vi "ProgressCmdResponse.vi"(6 "error in (no error)":errorcluster, 8 "FW Message Length":i32, 9 "FW Message ID":i32, 10 "Command for FW upgrade":string="1||1||1||AC.bin||PC.bin||SC.bin", 11 "connection ID control":refnum<k5>) -> (0 "data out":string, 1 "error out":errorcluster, 3 "connection ID":refnum<k5>)   [LabVIEW 2017]
panel:
  out "bytes written":i32
  # "Input"
  # "For Info:\nAC=1 Upgrade required, 0 Upgrade not required\nPC=1 Upgrade required, 0 Upgrade not required\nSC=1 Upgrade required, 0 Upgrade not required"
  # "Output"
  # "Refrence:"
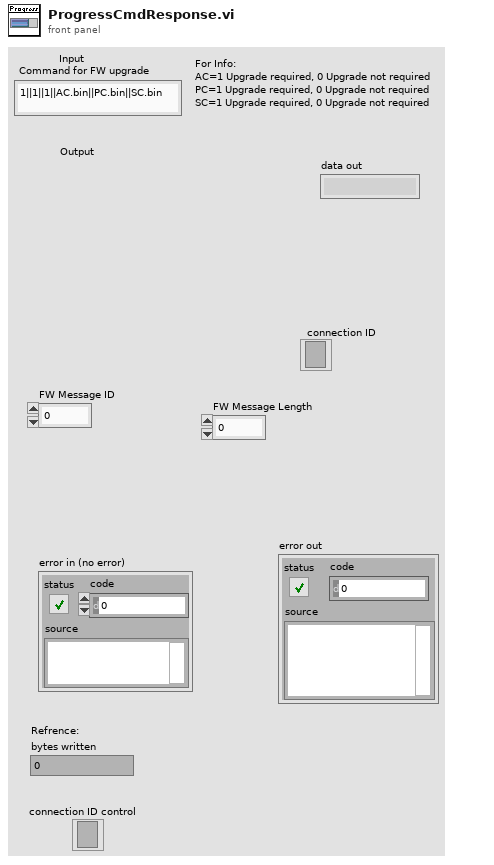
[diagram p1: front panel]
types:
  T1 = enum16{"big-endian, network order", "native, host order", "little-endian"}
  T2 = cluster{"FW Message Length":i32, "FW Message ID":i32}
  T3 = enum16{"Standard", "Buffered", "CRLF", "Immediate"}
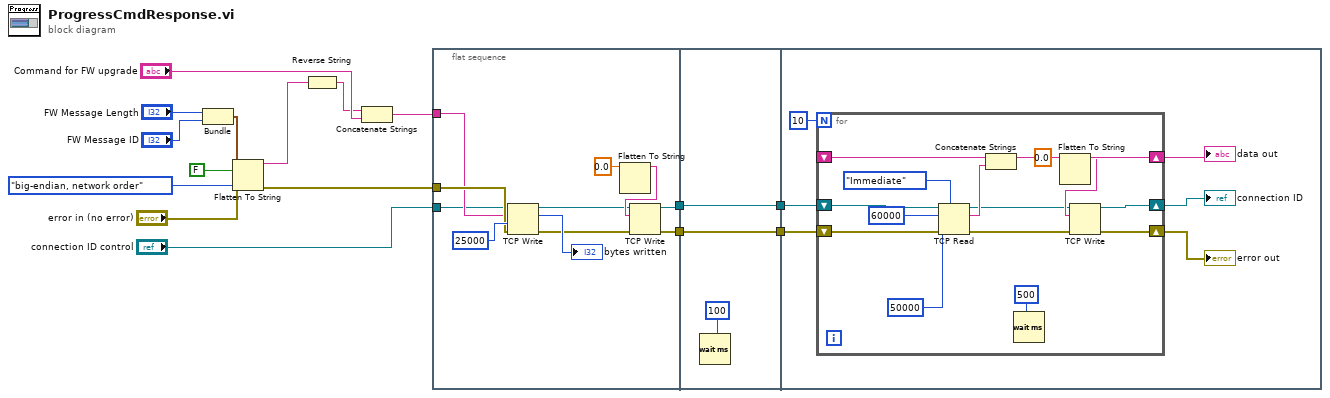
[diagram p0: block diagram]
diagram:
  n1 = Bundle("FW Message Length"="FW Message Length", "FW Message ID"="FW Message ID") -> (w10:T2)  [unwired: 1 in]
  n2 = Flatten To String(anything=w10, prepend array or string size? (T)=FALSE, byte order (0:big-endian, network order)=T1."big-endian, network order", error in (no error)="error in (no error)") -> (data string=w7:string, error out=w12:errorcluster)  [unwired: 1 out]
  n3 = Reverse String(1:w7) -> (0:w1:string)
  n4 = Concatenate Strings(w1, "Command for FW upgrade") -> (w6:string)
  n5 = flat-sequence {
    tunnel: [w18] -> w16
    tunnel: [w17] -> w15
    tunnel: w12 -> [w25]
    tunnel: w6 -> [w24]
    tunnel: "connection ID control" -> [w23]
    tunnel: w16 -> [w29]
    tunnel: w15 -> [w28]
    tunnel: [w29] -> w3
    tunnel: [w28] -> w2
    tunnel: w3 -> [w36]
    tunnel: w2 -> [w35]
    frame #0 {
      n6 = TCP Write(connection ID=w23, data in=w24, error in (no error)=w25, 9:25000 ("timeout ms (25000)")) -> (connection ID out=w19:refnum<k5>, bytes written=→"bytes written":i32, error out=w20:errorcluster)
      n7 = Flatten To String(anything=0.0) -> (data string=w21:string)  [unwired: 3 in, 2 out]
      n8 = TCP Write(connection ID=w19, data in=w21, error in (no error)=w20) -> (connection ID out=w18:refnum<k5>, error out=w17:errorcluster)  [unwired: 1 in, 1 out]
    }
    frame #1 {
      n9 = Wait (ms)(milliseconds to wait=u32 100) -> ()  [unwired: 1 out]
    }
    frame #2 {
      n10 = for {
        N: 10 -> [_]
        shift-right: [w39] -> w33
        shift-left: w36 -> [w51]
        shift-right: [w38] -> w34
        shift-left: w35 -> [w50]
        shift-right: [w44] -> w32
        shift-left: _ -> [w46]
        n11 = TCP Read(connection ID=w51, bytes to read=60000, error in (no error)=w50, 7:T3."Immediate" ("mode (standard)"), 9:50000 ("timeout ms (25000)")) -> (connection ID out=w40:refnum<k5>, data out=w45:string, error out=w41:errorcluster)
        n12 = Concatenate Strings(w46, w45) -> (w44:string)
        n13 = Wait (ms)(milliseconds to wait=u32 500) -> ()  [unwired: 1 out]
        n14 = Flatten To String(anything=0.0) -> (data string=w42:string)  [unwired: 3 in, 2 out]
        n15 = TCP Write(connection ID=w40, data in=w42, error in (no error)=w41) -> (connection ID out=w39:refnum<k5>, error out=w38:errorcluster)  [unwired: 1 in, 1 out]
      }
      "error out" <- w34
      "connection ID" <- w33
      "data out" <- w32
    }
  }
